vi "Launch Session.vi"(8 "error in (no error)":errorcluster) -> (0 "error out":errorcluster, 3 "Unit Of Work out":refnum<class "Unit Of Work Session.lvclass">)   [LabVIEW 2020, in "Conditu2.lvlib" / "Unit Of Work Session.lvclass"]
uses:
  Unit Of Work Session.lvclass
  Daemon Async.vi
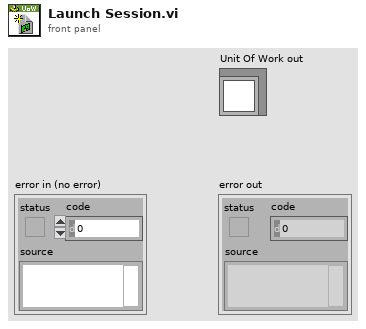
[diagram p1: front panel]
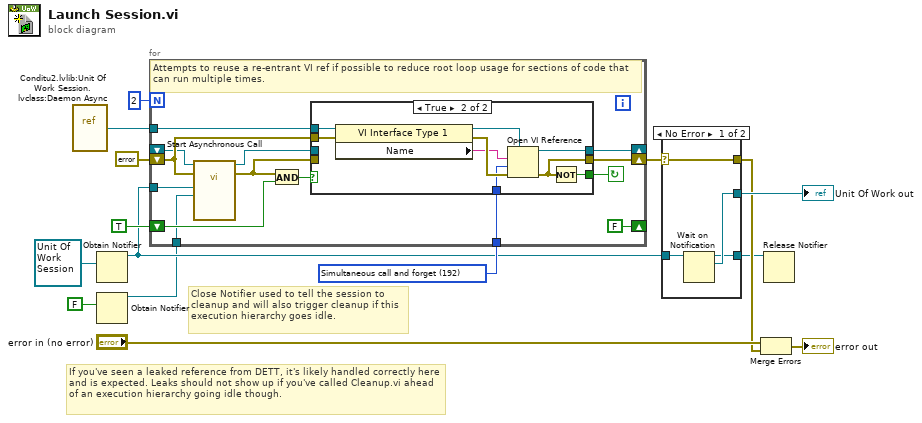
[diagram p0: block diagram]
diagram:
  w14 = 192 items=["Record modifications"=1, "Open templates for editing"=2, "Prompt user to save"=4, "Prepare for reentrant run"=8, "Prompt to find missing subVIs"=16, "Hide loading dialog box"=32, "Enable simultaneous calls"=64, "Prepare to call and forget"=128, "Simultaneous call and forget"=192, "Prepare to call and collect"=256, "Simultaneous call and collect"=320]
  # "If you've seen a leaked reference from DETT, it's likely handled correctly here and is expected. Leaks should not show up if you've called Cleanup.vi ahead of an execution hierarchy going idle though."
  # "Close Notifier used to tell the session to cleanup and will also trigger cleanup if this execution hierarchy goes idle."
  n1 = vi-ref "Conditu2.lvlib:Unit Of Work Session.lvclass:Daemon Async.vi"() -> (w15:refnum<vi>)
  n2 = Obtain Notifier(notification data type=refnum<class "Unit Of Work Session.lvclass"> refnum ("Conditum:Unit Of Work")) -> (notifier out=w9:refnum<notifier>)  [unwired: 3 in, 2 out]
  n3 = Obtain Notifier(notification data type=FALSE) -> (notifier out=w2:refnum<notifier>)  [unwired: 3 in, 2 out]
  n4 = for {
    N: 2 -> [_]
    tunnel: w15 -> [w28]
    tunnel: w14 -> [w27]
    shift-right: [w26] -> _
    shift-left: _ -> [w25]
    shift-right: [w23] -> w10
    shift-left: errorcluster {"status"=FALSE, "code"=0, "source"=""} ("error constant") -> [w29]
    shift-right: [FALSE] -> _
    shift-left: TRUE -> [w20]
    tunnel: w9 -> [w17]
    tunnel: w2 -> [w16]
    stop <- w19 continue-if-true
    # "Attempts to reuse a re-entrant VI ref if possible to reduce root loop usage for sections of code that can run multiple times."
    n5 = call-by-ref "Start Asynchronous Call"(reference=w25, error in=w29, "Close Notifier"=w16, "Session Notifier"=w17) -> (reference out=w24:refnum<vi>, error out=w22:errorcluster)  [unwired: 10 in]
    n6 = And(x=w22, y=w20) -> (x .and. y?=w21:bool)
    n7 = case shown="True" w21 {
      tunnel: w28 -> [_ w39]
      tunnel: w27 -> [_ w37]
      tunnel: [w31 w35] -> w26
      tunnel: w24 -> [w31 _]
      tunnel: [w30 w33] -> w23
      tunnel: w22 -> [w30 _]
      tunnel: w29 -> [_ w34]
      tunnel: [_ w32] -> w19
      frame False {
      }
      frame True {
        n8 = property class="VI Interface Type 1"(reference=w39, error in=w34) -> (reference out=w36:refnum<vi>, error out=w40:errorcluster, "Name"=w38:string)
        n9 = Open VI Reference(type specifier VI Refnum (for type only)=w36, vi path=w38, options=w37, error in (no error)=w40) -> (vi reference=w35:refnum<vi>, error out=w33:errorcluster)  [unwired: 2 in]
        n10 = Not(x=w33) -> (.not. x?=w32:bool)
      }
    }
  }
  n11 = case shown="No Error" w10 {
    selector: w10 -> [w43 w46]
    tunnel: w9 -> [w44 w45]
    tunnel: [w42 _] -> w8
    tunnel: [w43 w46] -> w6
    tunnel: [w41 w45] -> w1
    frame No Error {
      n12 = Wait on Notification(notifier=w44) -> (notifier out=w41:refnum<notifier>, notification=w42:refnum<class "Unit Of Work Session.lvclass">)  [unwired: 3 in, 2 out]
    }
    frame Error {
    }
  }
  "Unit Of Work out" <- w8
  n13 = Merge Errors("error in (no error)", w6) -> (→"error out":errorcluster)
  n14 = Release Notifier(notifier=w1) -> ()  [unwired: 2 in, 3 out]
